vi "Set Variables.vi"(8 "error in (no error)":errorcluster, 10 "Variables":variant, 11 "For Loop in":refnum<class "While Loop.lvclass">) -> (0 "error out":errorcluster, 3 "For Loop out":refnum<class "While Loop.lvclass">)   [LabVIEW 2016, in "While Loop.lvclass"]
uses:
  While Loop.lvclass
  While Loop.lvclass/While Loop.ctl
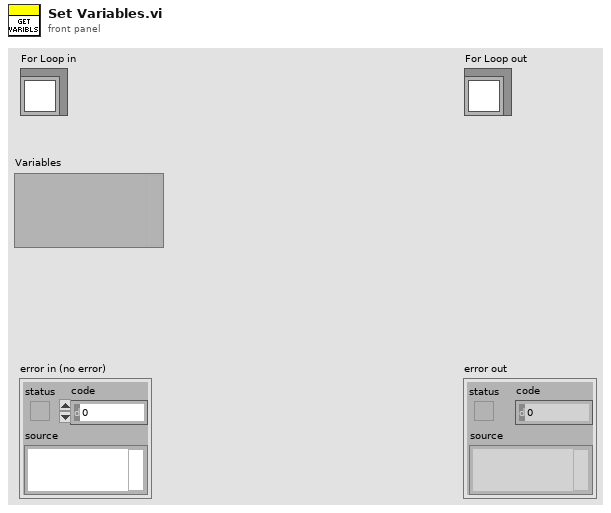
[diagram p1: front panel]
types:
  T1 = typedef "While Loop.lvclass/Variables.ctl" = cluster{"Continue?":bool}
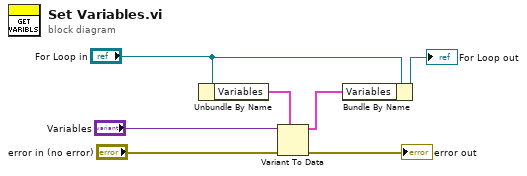
[diagram p0: block diagram]
diagram:
  n1 = Unbundle By Name("For Loop in") -> ("Variables"=w2:T1)
  n2 = Variant To Data(error in="error in (no error)", type=w2, Variant="Variables") -> (data=w1:T1, error out=→"error out":errorcluster)
  n3 = Bundle By Name(cluster="For Loop in", "Variables"=w1) -> (→"For Loop out":refnum<class "While Loop.lvclass">)
